vi "Actor.vi"(10 "Config Actor":T1, 11 "TEMPLATE Actor in":refnum<class "TEMPLATE Actor.lvclass">) -> (0 "Error out":errorcluster, 3 "TEMPLATE Actor out":refnum<class "TEMPLATE Actor.lvclass">)   [LabVIEW 2025, in "_Template.lvlib" / "Templates.lvlib" / "TEMPLATE Actor.lvlib" / "TEMPLATE Actor.lvclass"]
uses:
  TEMPLATE Actor.lvclass
  jettl/jettl/Actor/Config Actor.ctl
  jettl/jettl/Attributes/Attributes/Attributes.lvclass
  Control Refs.ctl
  TEMPLATE Actor.lvclass/TEMPLATE Actor.ctl
  jettl/jettl/Actor/Actor.lvlib
types:
  T1 = typedef "jettl.lvlib/Actor.lvlib/Config Actor.ctl" = cluster{"Alias":string, "Creator Attributes":refnum<class "Attributes.lvclass">, "Queue of Self Attributes":refnum<queue>, "Queue of Error":refnum<queue>}
  T2 = typedef "_Template.lvlib/Templates.lvlib/TEMPLATE Actor.lvlib/TEMPLATE Actor.lvclass/Control Refs.ctl" = cluster{"Placeholder":refnum<vi>}
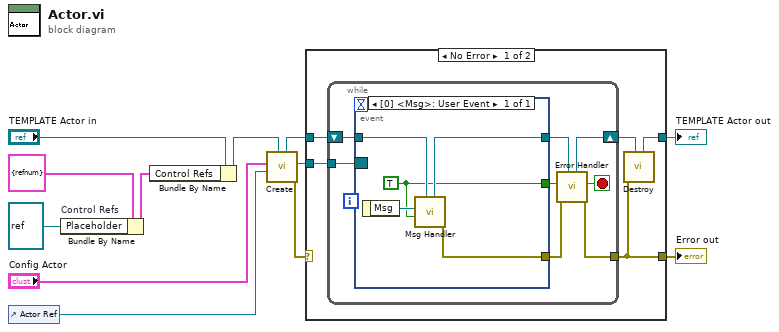
[diagram p0: block diagram]
diagram:
  n1 = control-ref of="Actor Ref"() -> (w1:refnum<vi>)
  n2 = Bundle By Name "Control Refs"(cluster=T2 {"Placeholder"=refnum} ("Process Refs"), "Placeholder"=refnum<vi> refnum) -> (w10:T2)
  n3 = Bundle By Name(cluster="TEMPLATE Actor in", "Control Refs"=w10) -> (w5:refnum<class "TEMPLATE Actor.lvclass">)
  n4 = call "Create.vi"("Actor in"=w5, "Actor Ref"=w1, "Config Actor"="Config Actor") -> ("Error out"=w6:errorcluster, "Event Ref"=w3:refnum<event-registration>, "Actor out"=w4:refnum<class "TEMPLATE Actor.lvclass">)  [unwired: 6 in]
  n5 = case shown="No Error" w6 {
    selector: w6 -> [_ w31]
    tunnel: [w13 w32] -> w12
    tunnel: w4 -> [w16 w32]
    tunnel: [w17 w31] -> w11
    tunnel: w3 -> [w15 _]
    frame No Error {
      n6 = while {
        shift-right: [w21] -> w14
        shift-left: w16 -> [w24]
        tunnel: w15 -> [w25]
        tunnel: [w22] -> w17
        stop <- w20 stop-if-true
        n7 = event shown="[0] <Msg>: User Event" {
          selector: w25 -> [_]
          dyn-events: _ -> [_]
          timeout: _ -> [_]
          tunnel: w24 -> [w28]
          tunnel: [w27] -> w19
          tunnel: [w30] -> w23
          tunnel: [w26] -> w18
          event User Event {
            w26 = TRUE ("From Msg Event")
            n8 = event-data() -> ("Msg"=w29:refnum<class "Msg.lvclass">)  [unwired: 1 in]
            n9 = call "Msg Handler.vi"("Actor in"=w28, "From Msg Event"=w26, "Msg"=w29) -> ("Error out"=w30:errorcluster, "Actor out"=w27:refnum<class "TEMPLATE Actor.lvclass">)  [unwired: 7 in]
          }
        }
        n10 = call "Error Handler.vi"("Actor in"=w19, "Error in"=w23, "From Msg Event"=w18) -> ("Error out"=w22:errorcluster, "Destroy"=w20:bool, "Actor out"=w21:refnum<class "TEMPLATE Actor.lvclass">)  [unwired: 6 in]
      }
      n11 = call "Destroy.vi"("Actor in"=w14, "Error in"=w17) -> ("Actor out"=w13:refnum<class "TEMPLATE Actor.lvclass">)  [unwired: 9 in]
    }
    frame Error {
    }
  }
  "TEMPLATE Actor out" <- w12
  "Error out" <- w11
